vi "CD Init_Get Status Channels Reference.vi"(8 "error in (no error)":errorcluster, 11 "Device Reference":T2 format="%.0x") -> (0 "error out":errorcluster, 3 "Array":T1[](array[typedef]) format="%.0x")   [LabVIEW 2019, in "Ballard Arinc-429 Engine.lvlib"]
doc: "This VI gets references for all Status Channels used."
uses:
  Ballard Arinc-429 Engine.lvlib
  <vilib>/NI VeriStand/Custom Device API/Custom Device Item Ref.ctl
  <vilib>/NI VeriStand/Custom Device API/Data Reference.ctl
  <vilib>/NI VeriStand/Custom Device API/Data Access Type.ctl
  Shared/Controls and Global/Global.vi
  <vilib>/NI VeriStand/Custom Device Tools/Custom Device Utility Library/NI VeriStand - Search for Item by GUID.vi
  <vilib>/NI VeriStand/Custom Device API/Custom Device API.lvlib
  Shared/Ballard Arinc-429 Shared.lvlib
  <vilib>/NI VeriStand/Custom Device Tools/Custom Device Utility Library/Custom Device Utility Library.lvlib
  System Explorer/Ballard Arinc-429 System Explorer.lvlib
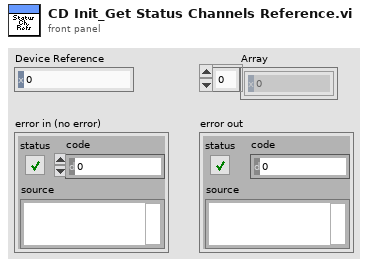
[diagram p1: front panel]
types:
  T1 = typedef "Custom Device API.lvlib/Data Reference.ctl" = i32
  T2 = typedef "Custom Device API.lvlib/Custom Device Item Ref.ctl" = u64
  T3 = typedef "Custom Device API.lvlib/Data Access Type.ctl" = enum16{"Read", "Write"}
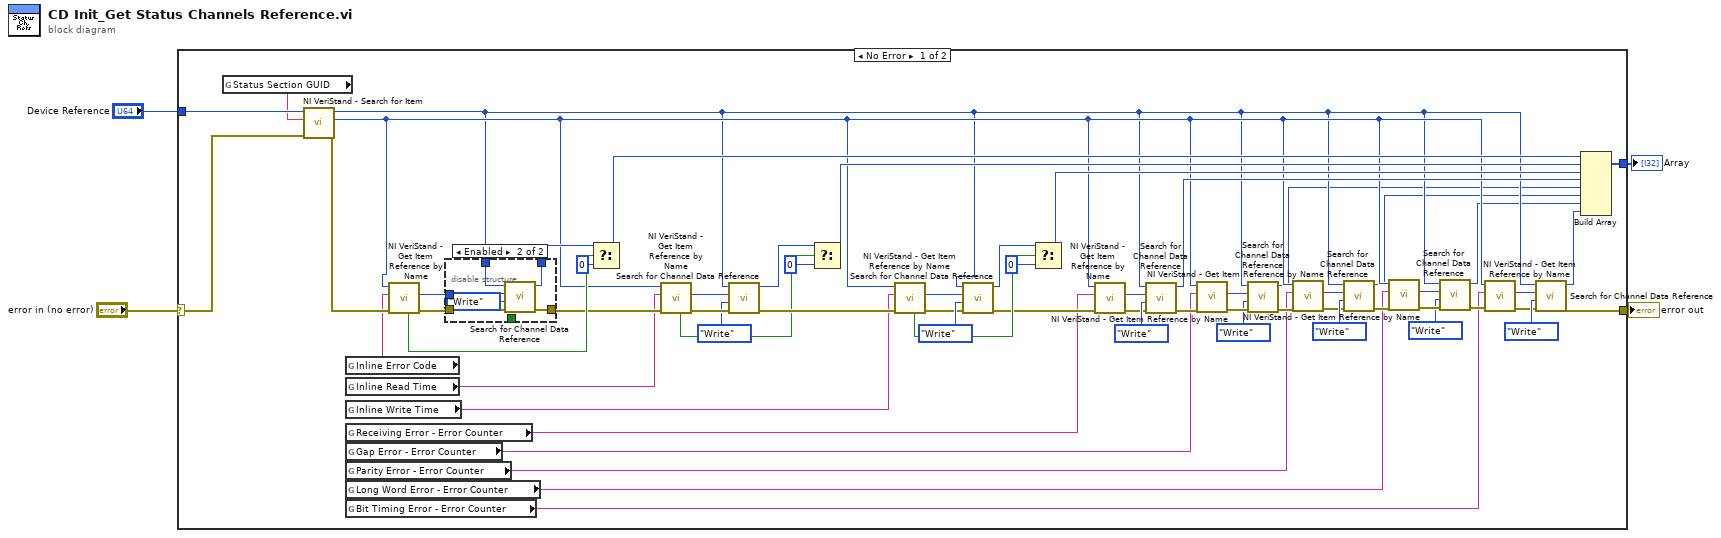
[diagram p0: block diagram]
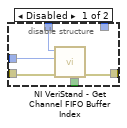
[diagram p2: hidden frame]
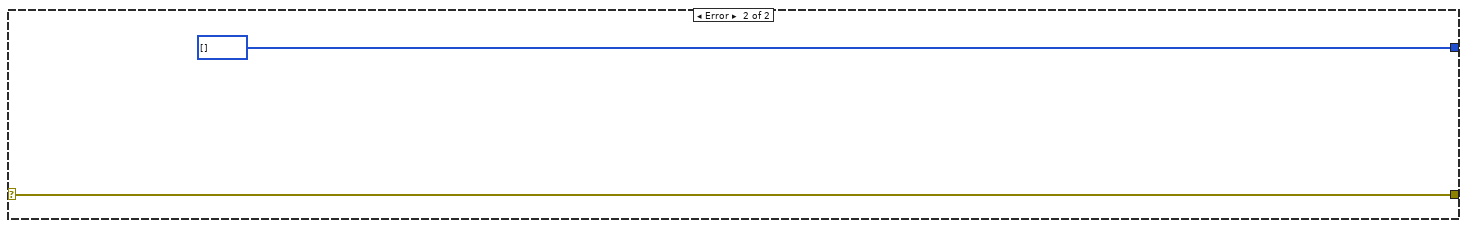
[diagram p3: hidden frame]
diagram:
  n1 = case shown="No Error" "error in (no error)" {
    selector: "error in (no error)" -> [w38 w80]
    tunnel: [w15 w80] -> w4
    tunnel: "Device Reference" -> [w47 _]
    tunnel: [w41 T1[] []] -> w2
    frame No Error {
      n2 = global read "Global.vi" "Status Section GUID"() -> (w46:string)
      n3 = call-poly <vilib>:"NI VeriStand - Search for Item.vi"("error in"=w38, "Item GUID"=w46, "Section Ref in"=w47) -> ("error out"=w51:errorcluster, "Item Ref"=w10:T2, "Section Ref out"=w9:T2)  [unwired: 5 in, 1 out]
      n4 = global read "Global.vi" "Inline Error Code"() -> (w42:string)
      n5 = global read "Global.vi" "Inline Read Time"() -> (w39:string)
      n6 = global read "Global.vi" "Inline Write Time"() -> (w65:string)
      n7 = global read "Global.vi" "Receiving Error - Error Counter"() -> (w36:string)
      n8 = global read "Global.vi" "Gap Error - Error Counter"() -> (w14:string)
      n9 = global read "Global.vi" "Parity Error - Error Counter"() -> (w13:string)
      n10 = global read "Global.vi" "Long Word Error - Error Counter"() -> (w12:string)
      n11 = global read "Global.vi" "Bit Timing Error - Error Counter"() -> (w11:string)
      n12 = call <vilib>:"NI VeriStand - Get Item Reference by Name.vi"("error in (no error)"=w51, "Item Name"=w42, "Parent Ref in"=w10) -> ("error out"=w44:errorcluster, "Item Ref"=w48:T2, "Found"=w50:bool)  [unwired: 5 in, 1 out]
      n13 = disable-structure shown="Enabled" {
        disable-tunnel: w44 -> [w72 w78]
        disable-tunnel: [w71 _] -> _
        disable-tunnel: [w70 w75] -> w45
        disable-tunnel: w9 -> [w69 w77]
        disable-tunnel: w48 -> [w68 w76]
        disable-tunnel: [_ w74] -> w49
        frame Disabled {
          n14 = call <vilib>:"NI VeriStand - Get Channel FIFO Buffer Index.vi"("error in"=w72, "Channel Ref"=w68, "Device Ref in"=w69) -> ("error out"=w70:errorcluster, "Found"=w71:bool)  [unwired: 4 in, 3 out]
        }
        frame Enabled {
          n15 = call "Search for Channel Data Reference.vi"("error in (no error)"=w78, "Access"=Data_Access_Type."Write", "Item Ref"=w76, "Device Ref in"=w77) -> ("error out"=w75:errorcluster, "Channel Data Reference"=w74:T1)  [unwired: 6 in]
        }
      }
      n16 = Select(t=w49, s=w50, f=T1 0) -> (s? t:f=w43:T1)
      n17 = call <vilib>:"NI VeriStand - Get Item Reference by Name.vi"("error in (no error)"=w45, "Item Name"=w39, "Parent Ref in"=w10) -> ("error out"=w54:errorcluster, "Item Ref"=w58:T2, "Found"=w55:bool)  [unwired: 5 in, 1 out]
      n18 = call "Search for Channel Data Reference.vi"("error in (no error)"=w54, "Access"=Data_Access_Type."Write", "Item Ref"=w58, "Device Ref in"=w9) -> ("error out"=w66:errorcluster, "Channel Data Reference"=w56:T1)  [unwired: 6 in]
      n19 = Select(t=w56, s=w55, f=T1 0) -> (s? t:f=w40:T1)
      n20 = call <vilib>:"NI VeriStand - Get Item Reference by Name.vi"("error in (no error)"=w66, "Item Name"=w65, "Parent Ref in"=w10) -> ("error out"=w63:errorcluster, "Item Ref"=w59:T2, "Found"=w62:bool)  [unwired: 5 in, 1 out]
      n21 = call "Search for Channel Data Reference.vi"("error in (no error)"=w63, "Access"=Data_Access_Type."Write", "Item Ref"=w59, "Device Ref in"=w9) -> ("error out"=w37:errorcluster, "Channel Data Reference"=w61:T1)  [unwired: 6 in]
      n22 = Select(t=w61, s=w62, f=T1 0) -> (s? t:f=w67:T1)
      n23 = call <vilib>:"NI VeriStand - Get Item Reference by Name.vi"("error in (no error)"=w37, "Item Name"=w36, "Parent Ref in"=w10) -> ("error out"=w33:errorcluster, "Item Ref"=w34:T2)  [unwired: 5 in, 2 out]
      n24 = call "Search for Channel Data Reference.vi"("error in (no error)"=w33, "Access"=Data_Access_Type."Write", "Item Ref"=w34, "Device Ref in"=w9) -> ("error out"=w28:errorcluster, "Channel Data Reference"=w32:T1)  [unwired: 6 in]
      n25 = call <vilib>:"NI VeriStand - Get Item Reference by Name.vi"("error in (no error)"=w28, "Item Name"=w14, "Parent Ref in"=w10) -> ("error out"=w31:errorcluster, "Item Ref"=w30:T2)  [unwired: 5 in, 2 out]
      n26 = call "Search for Channel Data Reference.vi"("error in (no error)"=w31, "Access"=Data_Access_Type."Write", "Item Ref"=w30, "Device Ref in"=w9) -> ("error out"=w24:errorcluster, "Channel Data Reference"=w5:T1)  [unwired: 6 in]
      n27 = call <vilib>:"NI VeriStand - Get Item Reference by Name.vi"("error in (no error)"=w24, "Item Name"=w13, "Parent Ref in"=w10) -> ("error out"=w25:errorcluster, "Item Ref"=w26:T2)  [unwired: 5 in, 2 out]
      n28 = call "Search for Channel Data Reference.vi"("error in (no error)"=w25, "Access"=Data_Access_Type."Write", "Item Ref"=w26, "Device Ref in"=w9) -> ("error out"=w20:errorcluster, "Channel Data Reference"=w6:T1)  [unwired: 6 in]
      n29 = call <vilib>:"NI VeriStand - Get Item Reference by Name.vi"("error in (no error)"=w20, "Item Name"=w12, "Parent Ref in"=w10) -> ("error out"=w23:errorcluster, "Item Ref"=w22:T2)  [unwired: 5 in, 2 out]
      n30 = call "Search for Channel Data Reference.vi"("error in (no error)"=w23, "Access"=Data_Access_Type."Write", "Item Ref"=w22, "Device Ref in"=w9) -> ("error out"=w16:errorcluster, "Channel Data Reference"=w7:T1)  [unwired: 6 in]
      n31 = call <vilib>:"NI VeriStand - Get Item Reference by Name.vi"("error in (no error)"=w16, "Item Name"=w11, "Parent Ref in"=w10) -> ("error out"=w17:errorcluster, "Item Ref"=w18:T2)  [unwired: 5 in, 2 out]
      n32 = call "Search for Channel Data Reference.vi"("error in (no error)"=w17, "Access"=Data_Access_Type."Write", "Item Ref"=w18, "Device Ref in"=w9) -> ("error out"=w15:errorcluster, "Channel Data Reference"=w8:T1)  [unwired: 6 in]
      n33 = Build Array(w43, w40, w67, w32, w5, w6, w7, w8) -> (w41:T1[])
    }
    frame Error {
    }
  }
  "error out" <- w4
  "Array" <- w2
